vi "AcquireDecayData.vi"() -> ()   [LabVIEW 2014]
uses:
  <vilib>/Platform/TimedLoop/XDataNode/timing_clust.ctl
  <vilib>/Platform/TimedLoop/XDataNode/nitl_modes.ctl
  <vilib>/Platform/TimedLoop/XDataNode/wakeup.ctl
  <vilib>/platform/TimedLoop/XDataNode/XDataNode.xnode
  <vilib>/Platform/TimedLoop/XDataNode/XDNodeRunTimeDep.lvlib
panel:
  out "Waveform Graph":i32[](graph)
  in  "Path":path
  in  "Acquisition Time (s)":dbl
  in  "Period (s)":dbl
  in  "stop":bool
  out "counts per second":dbl(knob) scale=0.0..100.0
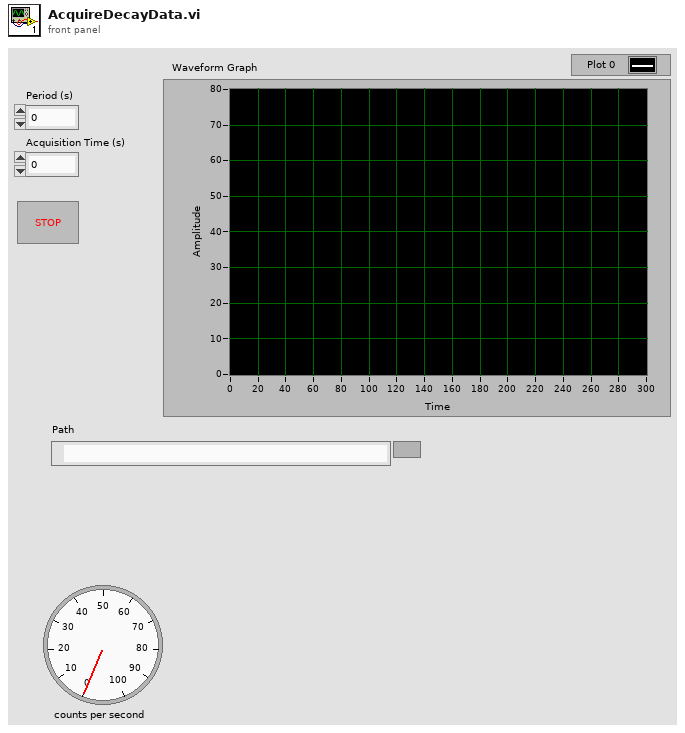
[diagram p1: front panel]
types:
  T1 = typedef "XDNodeRunTimeDep.lvlib/timing_clust.ctl" = cluster{"Expected End [f-1]":u64, "Actual End [f-1]":u64, "Finished Late? [f-1]":bool, "Expected End [i-1]":u64, "Actual End [i-1]":u64, "Finished Late? [i-1]":bool, "Expected Start [i]":u64, "Actual Start [i]":u64, "Expected Start [f]":u64, "Actual Start [f]":u64, "Source Name":string, "Structure Name":string, "Period":i64, "Deadline":i64, "Offset":i64, "Start":i64, "Priority":i32, "Timeout":i32, "Mode":T2, "Wakeup Reason":T3, "Error":errorcluster, "Source Type":string, "Secondary Source Type":string, "Global End Time":u64, "Global Start Time":u64, "Frame Duration":u64, "Iteration Duration":u64, "Assigned CPU":i32, "I/O Scan Engine Mode":u32}
  T2 = typedef "XDNodeRunTimeDep.lvlib/nitl_modes.ctl" = enum32{"No Change", "Process missed periods, maintain original phase", "Discard missed periods, maintain original phase", "Process missed periods, ignore original phase", "Discard missed periods, ignore original phase"}
  T3 = typedef "XDNodeRunTimeDep.lvlib/wakeup.ctl" = enum32{"Normal", "Aborted", "Asynchronous wakeup", "Timing source error", "Timed loop error", "Timeout"}
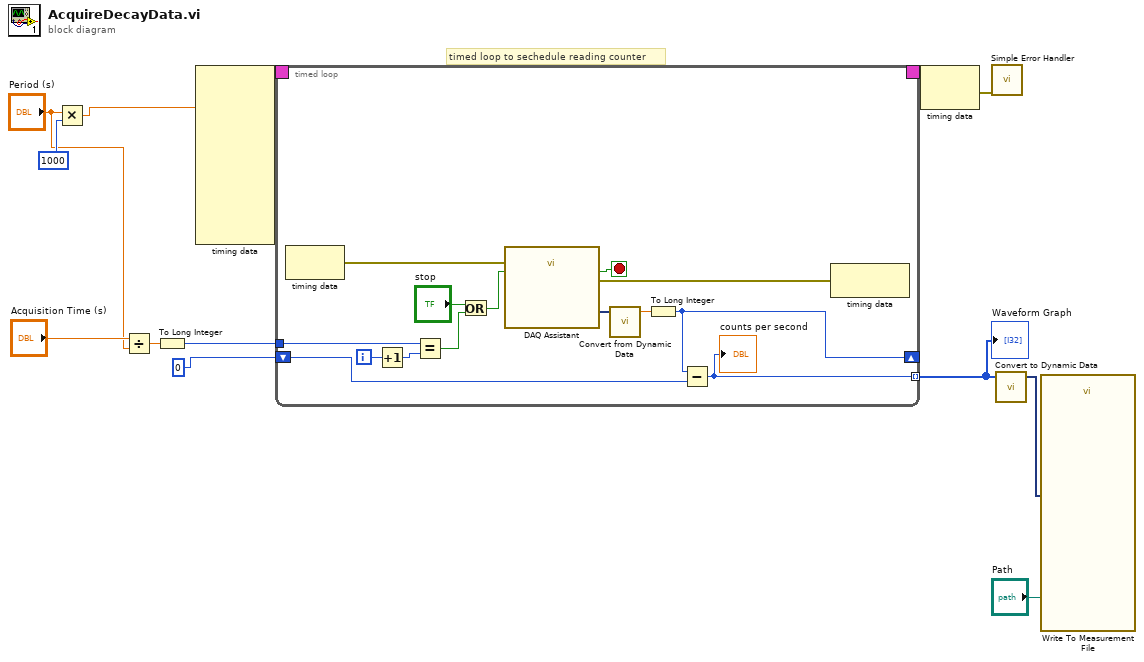
[diagram p0: block diagram]
diagram:
  # "timed loop to sechedule reading counter"
  n1 = Multiply(x="Period (s)", y=1000) -> (x*y=w2:dbl)
  n2 = Divide(x="Acquisition Time (s)", y="Period (s)") -> (x/y=w8:dbl)
  n3 = To Long Integer(number=w8) -> (32bit integer=w7:i32)
  n4 = node-c288(w2) -> (w13:T1)  [unwired: 9 in]
  n5 = timed-loop {
    timing: w13 -> [_]
    timing-out: [_] -> w12
    shift-right: [w24] -> _
    shift-left: 0 -> [w26]
    tunnel: w7 -> [w20]
    tunnel: [w14] -> w5 mode=indexing
    i -> [w19]
    stop <- w25 stop-if-true
    n6 = node-c288() -> (w21:errorcluster)  [unwired: 1 in]
    n7 = Increment(x=w19) -> (x+1=w18:i32)
    n8 = Equal?(x=w20, y=w18) -> (x = y?=w17:bool)
    n9 = Or(x="stop", y=w17) -> (x .or. y?=w15:bool)
    n10 = call "DAQ Assistant"("error in"=w21, "stop (F)"=w15) -> ("data"=w27:dynamicdata, "stopped"=w25:bool, "error out"=w22:errorcluster)  [unwired: 14 in, 1 out]
    n11 = call "Convert from Dynamic Data"("Dynamic Data Type"=w27) -> ("Scalar"=w23:dbl)  [unwired: 3 in]
    n12 = To Long Integer(number=w23) -> (32bit integer=w24:i32)
    n13 = Subtract(x=w24, y=w26) -> (x-y=w14:i32)
    "counts per second" <- w14
    n14 = node-c288(w22) -> ()  [unwired: 1 out]
  }
  "Waveform Graph" <- w5
  n15 = node-c288(w12) -> (w10:errorcluster)
  n16 = call <vilib>:"Simple Error Handler.vi"("error in (no error)"=w10) -> ()  [unwired: 4 in, 5 out]
  n17 = call "Convert to Dynamic Data"("Array"=w5) -> ("Dynamic Data Type"=w4:dynamicdata)  [unwired: 3 in]
  n18 = call "Write To Measurement File"("Signals"=w4, "Filename"="Path") -> ()  [unwired: 15 in, 3 out]
